vi "Numeric Keyboard Setup.vi"(6 "Password Display (F)":bool, 7 "Message In":string, 9 "String In":string, 10 "Max Length (50)":i32=50, 11 "String in":refnum<vi>) -> (0 "error out":errorcluster, 3 "String Out":string)   [LabVIEW 2015, in "Touch_keyboard.lvlib"]
doc: "This VI sets up the numeric keyboard front panel"
uses:
  Touch_keyboard.lvlib
  Driver Commands.ctl
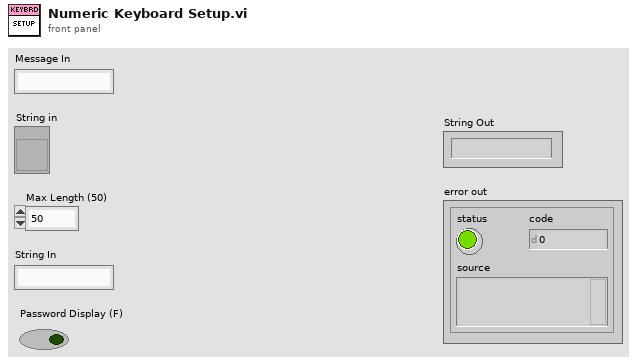
[diagram p1: front panel]
types:
  T1 = typedef "Touch_keyboard.lvlib/Driver Commands.ctl" = enum16{"No Command", "Initialize", "Add Character", "Replace Charcter", "Delete Character", "Move Left", "Move Right", "Update Edit Position"}
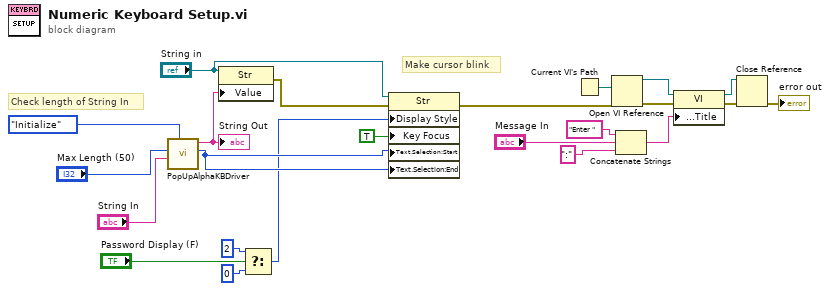
[diagram p0: block diagram]
diagram:
  # "Make cursor blink"
  # "Check length of String In"
  n1 = call "PopUpAlphaKBDriver.vi"("Driver Commands"=Driver_Commands."Initialize", "Initial String"="String In", "Max Length (70)"="Max Length (50)") -> ("Edit Position"=w11:i32, "String Out"=w12:string)  [unwired: 7 in]
  "String Out" <- w12
  n2 = property class="Str"(reference="String in", "Value"=w12) -> (error out=w2:errorcluster)  [unwired: 1 in, 1 out]
  n3 = Select(t=u32 2 ("Display Style"), s="Password Display (F)", f=u32 0 ("Display Style")) -> (s? t:f=w8:u32)
  n4 = property on="Property Node" class="Str"(reference="String in", error in=w2, "Display Style"=w8, "Key Focus"=TRUE, "Text.Selection:Start"=w11, "Text.Selection:End"=w11) -> (error out=w1:errorcluster)  [unwired: 1 out]
  n5 = Current VI's Path() -> (path=w19:path)
  n6 = Open VI Reference(vi path=w19, error in (no error)=w1) -> (vi reference=w18:refnum<vi>, error out=w17:errorcluster)  [unwired: 4 in]
  n7 = Concatenate Strings("Enter ", "Message In", ":" ("Substring")) -> (w14:string)
  n8 = property class="VI"(reference=w18, error in=w17, "Front Panel Window:Title"=w14) -> (reference out=w16:refnum<vi>, error out=w15:errorcluster)
  n9 = Close Reference(reference=w16, error in (no error)=w15) -> (error out=→"error out":errorcluster)
